vi "Gamepad Speed Drive.vi"(0 "Drive Powers":cluster{"Linear":dbl, "Turn":dbl}, 1 "Quick Turn":bool) -> (2 "Left Output":dbl, 3 "Right Output":dbl)   [LabVIEW 2014]
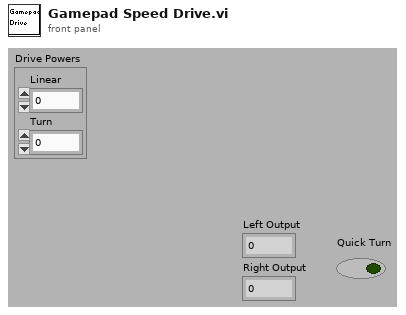
[diagram p1: front panel]
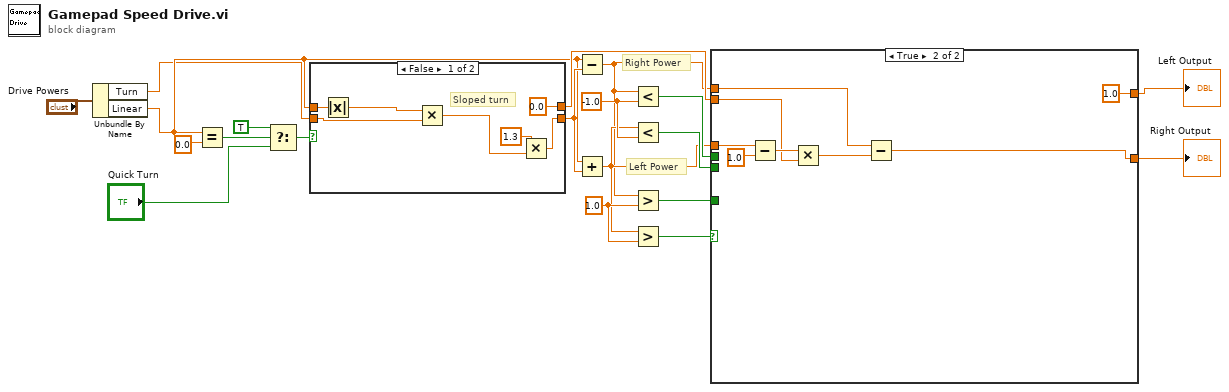
[diagram p0: block diagram]
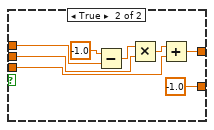
[diagram p3: hidden frame]
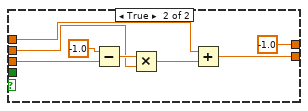
[diagram p4: hidden frame]
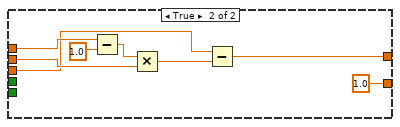
[diagram p5: hidden frame]
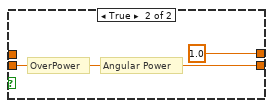
[diagram p6: hidden frame]
diagram:
  w15 = -1.0 ("y")
  w18 = 1.0 ("y")
  # "Right Power"
  # "Left Power"
  n1 = Unbundle By Name("Drive Powers") -> ("Turn"=w1:dbl, "Linear"=w2:dbl)
  n2 = Equal?(x=w2, y=0.0) -> (x = y?=w7:bool)
  n3 = Select(t=TRUE, s=w7, f="Quick Turn") -> (s? t:f=w6:bool)
  n4 = case shown="False" w6 {
    tunnel: w1 -> [w25 w28]
    tunnel: w2 -> [w27 _]
    tunnel: [0.0 1.0] -> w12
    tunnel: [w22 w28] -> w20
    frame False {
      # "Sloped turn"
      n5 = Absolute Value(x=w27) -> (abs(x)=w26:dbl)
      n6 = Multiply(x=w26, y=w25) -> (x*y=w24:dbl)
      n7 = Multiply(x=1.3 ("Numeric"), y=w24) -> (x*y=w22:dbl)
    }
    frame True {
      # "Angular Power"
      # "OverPower"
    }
  }
  n8 = Subtract(x=w2, y=w20) -> (x-y=w11:dbl)
  n9 = Add(x=w2, y=w20) -> (x+y=w13:dbl)
  n10 = Less?(x=w11, y=w15) -> (x < y?=w14:bool)
  n11 = Less?(x=w13, y=w15) -> (x < y?=w16:bool)
  n12 = Greater?(x=w11, y=w18) -> (0:w17:bool)
  n13 = Greater?(x=w13, y=w18) -> (0:w19:bool)
  n14 = case shown="True" w19 {
    tunnel: w17 -> [w37 _]
    tunnel: w16 -> [w36 _]
    tunnel: w14 -> [w35 _]
    tunnel: w13 -> [w31 w84]
    tunnel: w12 -> [w32 w81]
    tunnel: w11 -> [w33 w79]
    tunnel: [w34 w78] -> w9
    tunnel: [w30 1.0] -> w10
    frame False {
      n15 = case shown="False" w37 {
        tunnel: w36 -> [w44 _]
        tunnel: w35 -> [w43 _]
        tunnel: [w39 1.0] -> w34
        tunnel: w33 -> [w40 w72]
        tunnel: w32 -> [w41 w71]
        tunnel: w31 -> [w42 w70]
        tunnel: [w38 w69] -> w30
        frame False {
          n16 = case shown="False" w44 {
            tunnel: w43 -> [w50 _]
            tunnel: w42 -> [w47 w67]
            tunnel: w41 -> [w48 w65]
            tunnel: w40 -> [w49 w63]
            tunnel: [w45 w62] -> w39
            tunnel: [w46 -1.0] -> w38
            frame False {
              n17 = case shown="False" w50 {
                tunnel: w49 -> [w51 w59]
                tunnel: w48 -> [_ w57]
                tunnel: w47 -> [w52 w55]
                tunnel: [w52 w54] -> w46
                tunnel: [w51 -1.0] -> w45
                frame False {
                }
                frame True {
                  n18 = Subtract(x=-1.0, y=w59) -> (x-y=w58:dbl)
                  n19 = Multiply(x=w58, y=w57) -> (x*y=w56:dbl)
                  n20 = Add(x=w56, y=w55) -> (x+y=w54:dbl)
                }
              }
            }
            frame True {
              n21 = Subtract(x=-1.0, y=w67) -> (x-y=w66:dbl)
              n22 = Multiply(x=w66, y=w65) -> (x*y=w64:dbl)
              n23 = Add(x=w63, y=w64) -> (x+y=w62:dbl)
            }
          }
        }
        frame True {
          n24 = Subtract(x=w72, y=1.0) -> (x-y=w75:dbl)
          n25 = Multiply(x=w75, y=w71) -> (x*y=w76:dbl)
          n26 = Subtract(x=w70, y=w76) -> (x-y=w69:dbl)
        }
      }
    }
    frame True {
      n27 = Subtract(x=w84, y=1.0) -> (x-y=w82:dbl)
      n28 = Multiply(x=w82, y=w81) -> (x*y=w80:dbl)
      n29 = Subtract(x=w79, y=w80) -> (x-y=w78:dbl)
    }
  }
  "Left Output" <- w10
  "Right Output" <- w9
